vi "InitGObj.vi"(0 "Stand":refnum<class "Stand.lvclass">, 11 "error in":errorcluster) -> (4 "Stand out":refnum<class "Stand.lvclass">, 15 "error out":errorcluster)   [LabVIEW 2019, in "Stand.lvclass"]
uses:
  Stand_class/Stand.lvclass
  D:/GIT H4000/H4000/src/Proccess_class/Proccess.lvclass
  Proccess_class/Proccess.lvclass/Proccess.ctl
  MessageAMC_class/MessageAMC.lvclass
  D:/GIT H4000/H4000/src/MessageInterface_class/MessageInterface.lvclass
  Sig_AI_class/Sig_AI.lvclass
  Stand_class/Stand.lvclass/Stand.ctl
  Sig_DI_Simple_class/Sig_DI_Simple.lvclass
  Proccess_class/Proccess.lvclass
  NeedleValve_class/NeedleValve.lvclass
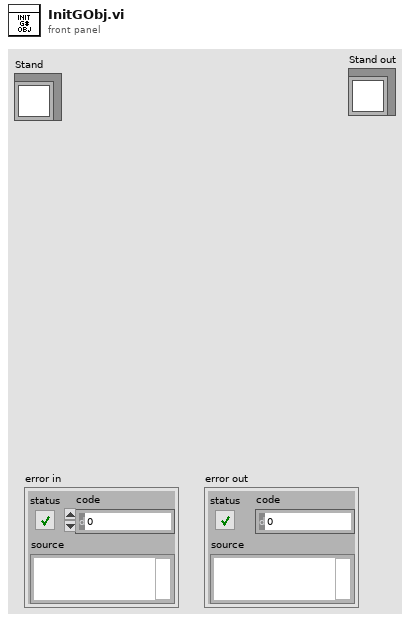
[diagram p1: front panel]
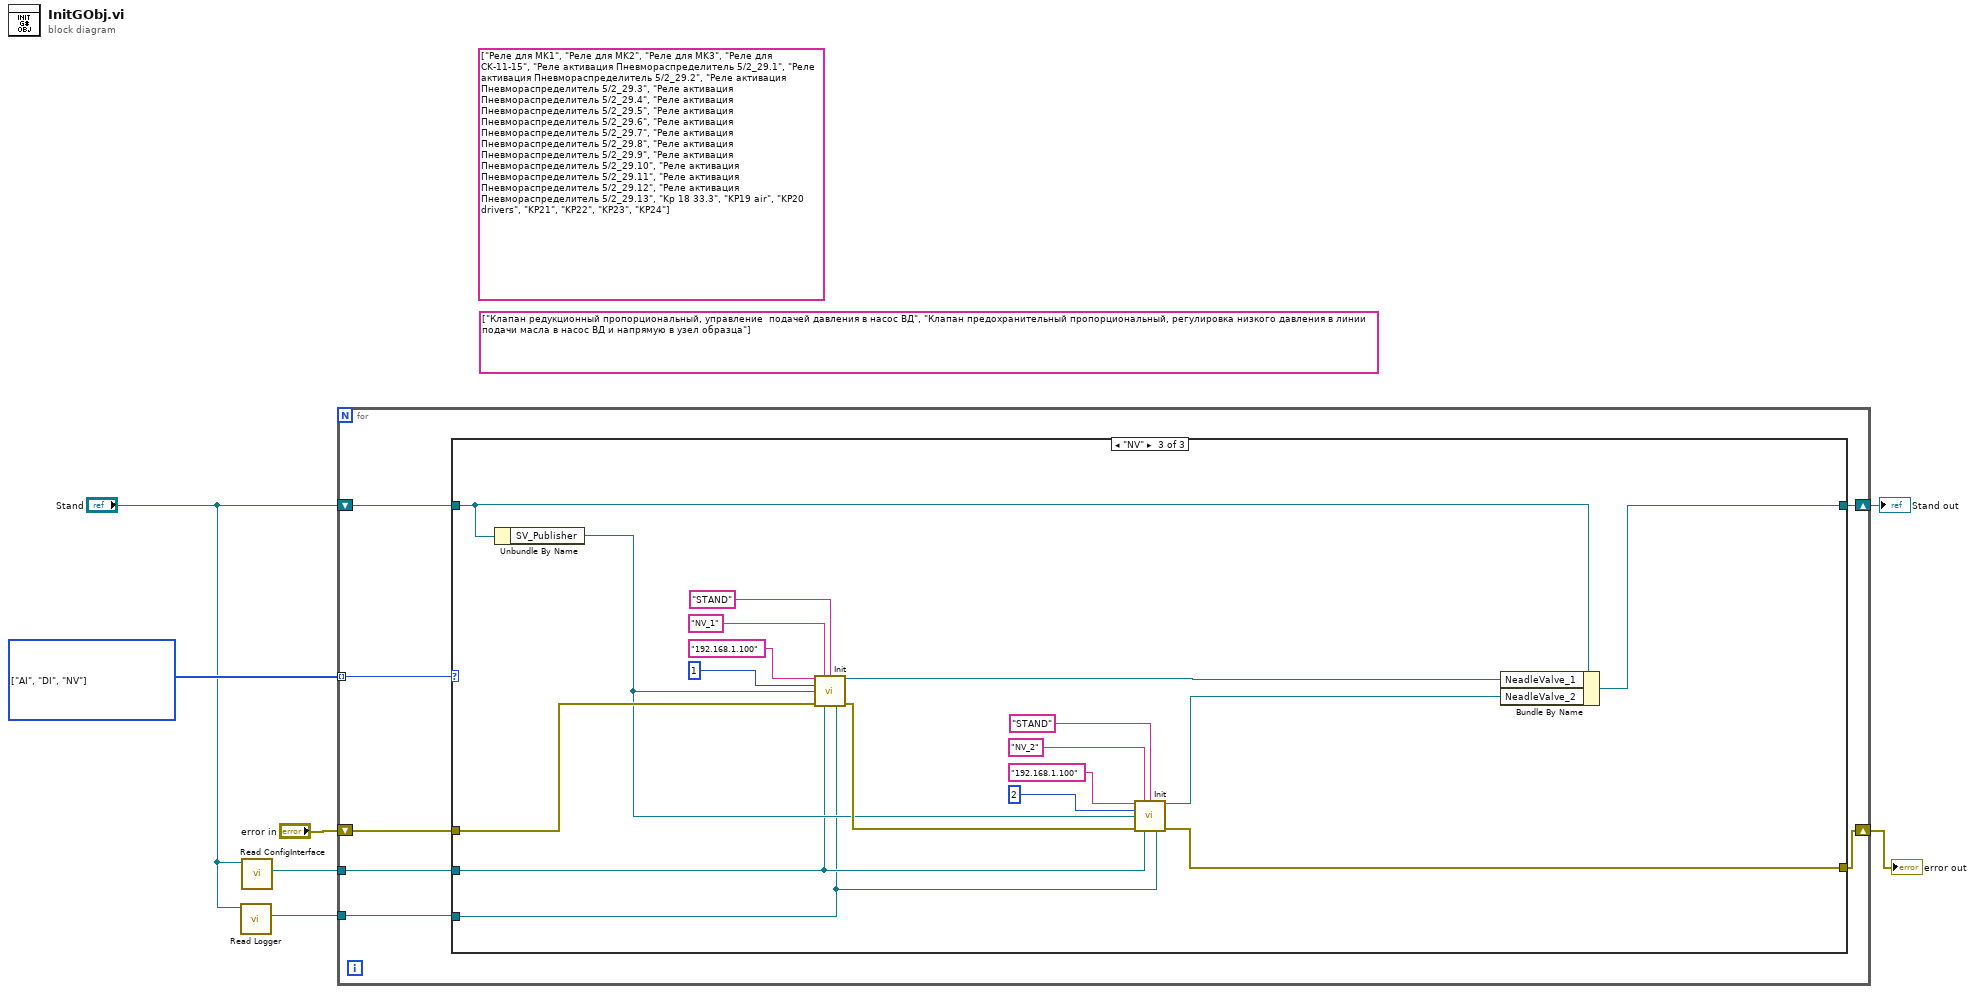
[diagram p0: block diagram]
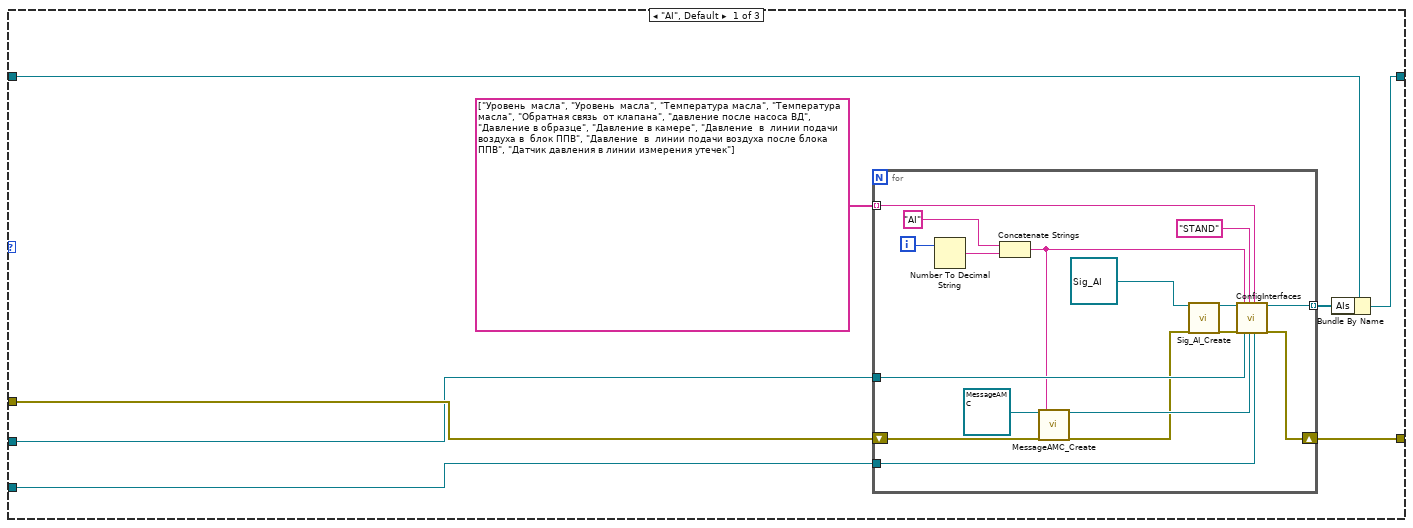
[diagram p2: hidden frame]
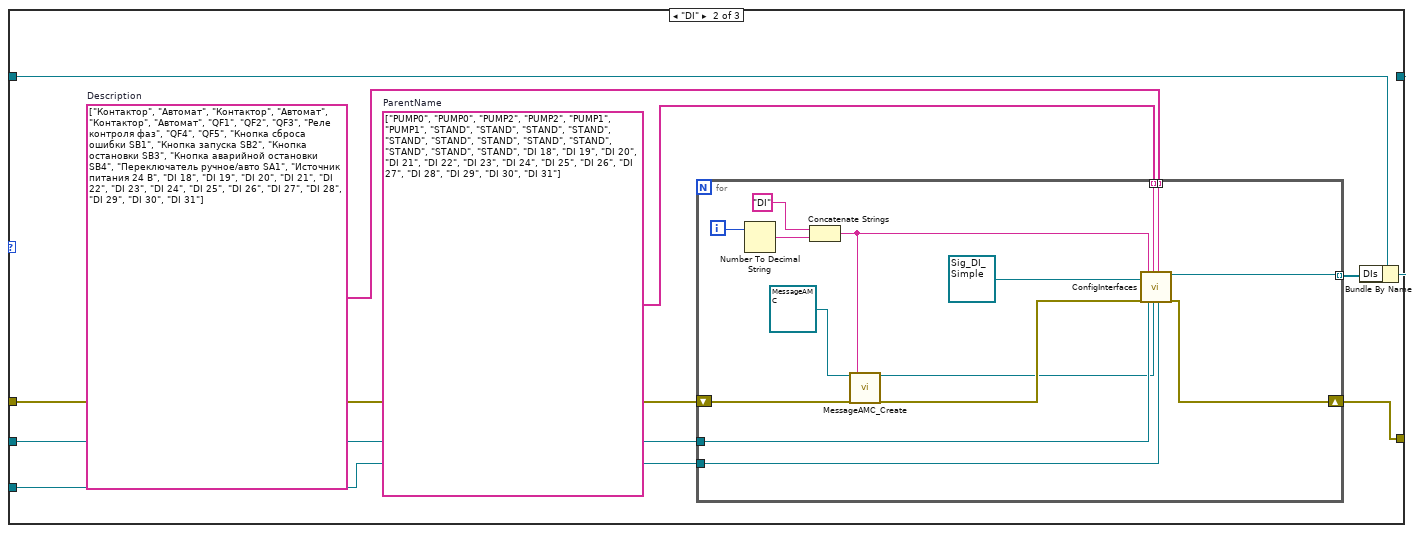
[diagram p3: hidden frame]
diagram:
  (unwired) string[] ["Реле для MK1", "Реле для MK2", "Реле для MK3", "Реле для CK-11-15", "Реле активация Пневмораспределитель 5/2_29.1", "Реле активация Пневмораспределитель 5/2_29.2", "Реле активация Пневмораспределитель 5/2_29.3", "Реле активация Пневмораспределитель 5/2_29.4", "Реле активация Пневмораспределитель 5/2_29.5", "Реле активация Пневмораспределитель 5/2_29.6", "Реле активация Пневмораспределитель 5/2_29.7", "Реле активация Пневмораспределитель 5/2_29.8", "Реле активация Пневмораспределитель 5/2_29.9", "Реле активация Пневмораспределитель 5/2_29.10", "Реле активация Пневмораспределитель 5/2_29.11", "Реле активация Пневмораспределитель 5/2_29.12", "Реле активация Пневмораспределитель 5/2_29.13", "Kp 18 33.3", "KP19 air", "KP20 drivers", "KP21", "KP22", "KP23", "KP24"] ("string array")
  (unwired) string[] ["Клапан редукционный пропорциональный, управление  подачей давления в насос ВД", "Клапан предохранительный пропорциональный, регулировка низкого давления в линии подачи масла в насос ВД и напрямую в узел образца"] ("ParentName")
  w7 = enum16{"AI", "DI", "NV"}[] [enum."AI", enum."DI", enum."NV"] items=["AI", "DI", "NV"]
  n1 = call "Read Logger.vi"("Proccess in"="Stand") -> ("Logger"=w3:refnum<class "Logger.lvclass">)  [unwired: 10 in]
  n2 = call "Read ConfigInterface.vi"("Proccess in"="Stand") -> ("ConfigInterface"=w1:refnum<class "ConfigInterface.lvclass">)  [unwired: 9 in, 1 out]
  n3 = for {
    tunnel: w3 -> [w14]
    tunnel: w7 -> [w13] mode=indexing
    shift-right: [w12] -> w5
    shift-left: "error in" -> [w11]
    shift-right: [w9] -> w4
    shift-left: "Stand" -> [w10]
    tunnel: w1 -> [w8]
    n4 = case shown="\"NV\"" w13 {
      tunnel: [w22 w44 w64] -> w12
      tunnel: w14 -> [w21 w42 w66]
      tunnel: w11 -> [w20 w47 w75]
      tunnel: w10 -> [w19 w48 w74]
      tunnel: [w18 w46 w81] -> w9
      tunnel: w8 -> [w16 w43 w67]
      frame "AI", Default {
        n5 = for {
          tunnel: [w33] -> w17 mode=indexing
          shift-right: [w34] -> w22
          shift-left: w20 -> [w36]
          tunnel: w21 -> [w29]
          tunnel: w16 -> [w30]
          tunnel: string[] ["Уровень  масла", "Уровень  масла", "Температура масла", "Температура масла", "Обратная связь  от клапана", "давление после насоса ВД", "Давление в образце", "Давление в камере", "Давление  в  линии подачи воздуха в  блок ППВ", "Давление  в  линии подачи воздуха после блока ППВ", "Датчик давления в линии измерения утечек"] ("ParentName") -> [w23] mode=indexing
          i -> [w39]
          n6 = Number To Decimal String(number=w39) -> (decimal integer string=w38:string)  [unwired: 1 in]
          n7 = Concatenate Strings("AI" ("string"), w38) -> (w24:string)
          n8 = call "MessageAMC_Create.vi"("reference in"=refnum<class "MessageAMC.lvclass"> refnum, "error in (no error)"=w36, "message queue name"=w24) -> ("amc"=w31:refnum<class "MessageAMC.lvclass">, "error out"=w25:errorcluster)  [unwired: 15 in]
          n9 = call "Sig_AI_Create.vi"("reference in"=refnum<class "Sig_AI.lvclass"> refnum ("Sig_AI"), "error in (no error)"=w25) -> ("reference out"=w27:refnum<class "Sig_AI.lvclass">, "error out"=w26:errorcluster)  [unwired: 16 in]
          n10 = call "ConfigInterfaces.vi"("reference in"=w27, "error in (no error)"=w26, "Name"=w24, "ConfigInterface"=w30, "ParentName"="STAND", "MessageInterface"=w31, "Description"=w23, "Logger"=w29) -> ("reference out"=w33:refnum<class "Sig_AI.lvclass">, "error out"=w34:errorcluster)  [unwired: 10 in]
        }
        n11 = Bundle By Name(cluster=w19, "AIs"=w17) -> (w18:refnum<class "Stand.lvclass">)
      }
      frame "DI" {
        w40 = string[] ["PUMP0", "PUMP0", "PUMP2", "PUMP2", "PUMP1", "PUMP1", "STAND", "STAND", "STAND", "STAND", "STAND", "STAND", "STAND", "STAND", "STAND", "STAND", "STAND", "STAND", "DI 18", "DI 19", "DI 20", "DI 21", "DI 22", "DI 23", "DI 24", "DI 25", "DI 26", "DI 27", "DI 28", "DI 29", "DI 30", "DI 31"]  # ParentName
        w41 = string[] ["Контактор", "Автомат", "Контактор", "Автомат", "Контактор", "Автомат", "QF1", "QF2", "QF3", "Реле контроля фаз", "QF4", "QF5", "Кнопка сброса ошибки SB1", "Кнопка запуска SB2", "Кнопка остановки SB3", "Кнопка аварийной остановки SB4", "Переключатель ручное/авто SA1", "Источник питания 24 В", "DI 18", "DI 19", "DI 20", "DI 21", "DI 22", "DI 23", "DI 24", "DI 25", "DI 26", "DI 27", "DI 28", "DI 29", "DI 30", "DI 31"]  # Description
        n12 = for {
          tunnel: [w57] -> w45 mode=indexing
          shift-right: [w56] -> w44
          shift-left: w47 -> [w59]
          tunnel: w43 -> [w54]
          tunnel: w42 -> [w55]
          tunnel: w41 -> [w51] mode=indexing
          tunnel: w40 -> [w50] mode=indexing
          i -> [w63]
          n13 = Number To Decimal String(number=w63) -> (decimal integer string=w62:string)  [unwired: 1 in]
          n14 = Concatenate Strings("DI" ("string"), w62) -> (w52:string)
          n15 = call "MessageAMC_Create.vi"("reference in"=refnum<class "MessageAMC.lvclass"> refnum, "error in (no error)"=w59, "message queue name"=w52) -> ("amc"=w53:refnum<class "MessageAMC.lvclass">, "error out"=w58:errorcluster)  [unwired: 15 in]
          n16 = call "ConfigInterfaces.vi"("reference in"=refnum<class "Sig_DI_Simple.lvclass"> refnum ("Sig_DI"), "error in (no error)"=w58, "Name"=w52, "ConfigInterface"=w54, "ParentName"=w50, "MessageInterface"=w53, "Description"=w51, "Logger"=w55) -> ("reference out"=w57:refnum<class "Sig_DI_Simple.lvclass">, "error out"=w56:errorcluster)  [unwired: 10 in]
        }
        n17 = Bundle By Name(cluster=w48, "DIs"=w45) -> (w46:refnum<class "Stand.lvclass">)
      }
      frame "NV" {
        n18 = Unbundle By Name(w74) -> ("SV_Publisher"=w68:refnum<class "SV_Publisher.lvclass">)
        n19 = call "Init.vi"("address"="192.168.1.100", "Name"="NV_1", "ParentName"="STAND", "addres"=u16 1, "SV_Publisher"=w68, "error in (no error)"=w75, "ConfigInterface"=w67, "Logger"=w66) -> ("NeedleValve out"=w76:refnum<class "NeedleValve.lvclass">, "error out"=w69:errorcluster)  [unwired: 6 in]
        n20 = call "Init.vi"("address"="192.168.1.100", "Name"="NV_2", "ParentName"="STAND", "addres"=u16 2, "SV_Publisher"=w68, "error in (no error)"=w69, "ConfigInterface"=w67, "Logger"=w66) -> ("NeedleValve out"=w65:refnum<class "NeedleValve.lvclass">, "error out"=w64:errorcluster)  [unwired: 6 in]
        n21 = Bundle By Name(cluster=w74, "NeadleValve_1"=w76, "NeadleValve_2"=w65) -> (w81:refnum<class "Stand.lvclass">)
      }
    }
  }
  "error out" <- w5
  "Stand out" <- w4
